vi "buildWorkerStopAll.vi"(8 "error in (no error)":errorcluster, 11 "BuildServer in":refnum<class "BuildServer.lvclass">) -> (0 "error out":errorcluster, 3 "BuildServer out":refnum<class "BuildServer.lvclass">)   [LabVIEW 2017, in "BuildServer.lvlib" / "BuildServer.lvclass"]
uses:
  BuildServer.lvclass
  BuildServer.lvclass/BuildServer.ctl
  Classes/BuildWorker Interface/BuildWorker/BuildWorker.lvclass
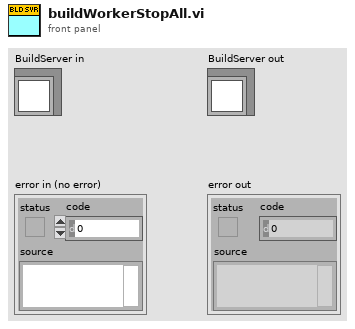
[diagram p1: front panel]
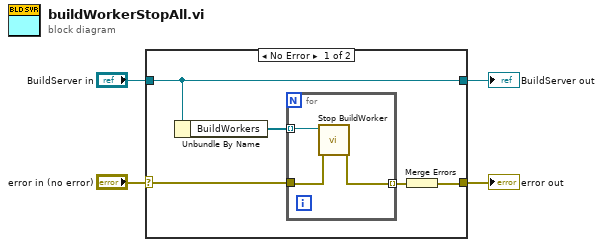
[diagram p0: block diagram]
diagram:
  n1 = case shown="No Error" "error in (no error)" {
    selector: "error in (no error)" -> [w7 w14]
    tunnel: [w5 w14] -> w3
    tunnel: [w9 w13] -> w1
    tunnel: "BuildServer in" -> [w9 w13]
    frame No Error {
      n2 = Unbundle By Name(w9) -> ("BuildWorkers"=w8:refnum<class "BuildWorker.lvclass">[])
      n3 = for {
        tunnel: w8 -> [w12] mode=indexing
        tunnel: [w10] -> w6 mode=indexing
        tunnel: w7 -> [w11]
        n4 = call "Stop BuildWorker.vi"("error in (no error)"=w11, "BuildWorker in"=w12) -> ("error out"=w10:errorcluster)  [unwired: 8 in, 1 out]
      }
      n5 = Merge Errors(w6) -> (w5:errorcluster)
    }
    frame Error {
    }
  }
  "error out" <- w3
  "BuildServer out" <- w1
